vi "PCO_SetTimeouts.vi"(8 "error in (no error)":errorcluster {"code" format="%x"}, 10 "buf_in":u32[](array[numeric])=[0, 0, 0], 11 "ph":u64) -> (0 "error out":errorcluster {"code" format="%x"}, 2 "ErrorMessage":i32 format="%x", 3 "ph out":u64)   [LabVIEW 2020, in "SDK.lvlib" / "GeneralCameraControl.lvlib"]
doc: "<b>Description:</b>\nThis function does set the internal timeout values for different tasks. Usually there is no need to change these values.\n\n<b>Supported camera type:</b>\nAll cameras\n\n<b>Descriptor dependency:</b>\nNone"
uses:
  GeneralCameraControl.lvlib
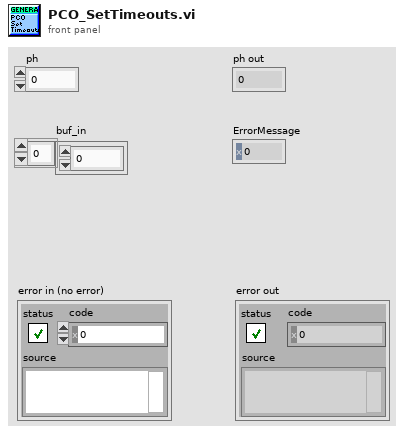
[diagram p1: front panel]
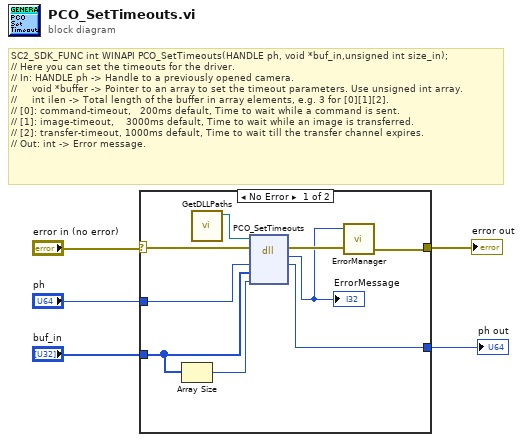
[diagram p0: block diagram]
diagram:
  # "SC2_SDK_FUNC int WINAPI PCO_SetTimeouts(HANDLE ph, void *buf_in,unsigned int size_in);\n// Here you can set the timeouts for the driver.\n// In: HANDLE ph -> Handle to a previously opened camera.\n//     void *buffer -> Pointer to an array to set the timeout parameters. Use unsigned int array.\n//     int ilen -> Total length of the buffer in array elements, e.g. 3 for [0][1][2].\n// [0]: command-timeout,   200ms default, Time to wait while a command is sent.\n// [1]: image-timeout,    3000ms default, Time to wait while an image is transferred.\n// [2]: transfer-timeout, 1000ms default, Time to wait till the transfer channel expires.\n// Out: int -> Error message."
  n1 = case shown="No Error" "error in (no error)" {
    selector: "error in (no error)" -> [w12 w16]
    tunnel: "ph" -> [w14 w15]
    tunnel: [w13 w15] -> w4
    tunnel: [w11 w16] -> w3
    tunnel: "buf_in" -> [w8 _]
    frame No Error {
      n2 = Array Size(array=w8) -> (size(s)=w7:i32)
      n3 = call "GetDLLPaths.vi"() -> ("SC2_Cam_Path"=w6:path)  [unwired: 9 in, 2 out]
      n4 = dll-call lib="?" fn="PCO_SetTimeouts"(path in=w6, error in=w12, "ph"=w14, "buf_in"=w8, "size_in"=w7) -> (error out=w10:errorcluster, "return type"=w9:i32, "ph"=w13:u64)  [unwired: 3 in, 1 out]
      "ErrorMessage" <- w9
      n5 = call "ErrorManager.vi"("error in (no error)"=w10, "error code"=w9) -> ("error out"=w11:errorcluster)  [unwired: 3 in]
    }
    frame Error {
    }
  }
  "ph out" <- w4
  "error out" <- w3
